vi "main.vi"() -> ()   [LabVIEW 2009]
panel:
  out "右表":dbl(knob) scale=0.0..100.0
  out "左表":dbl(knob) scale=0.0..100.0
  in  "右表旋转一圈":bool
  in  "stop":bool
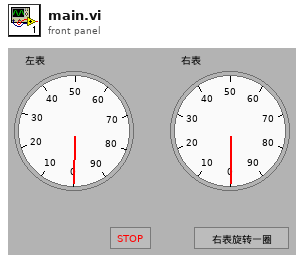
[diagram p1: front panel]
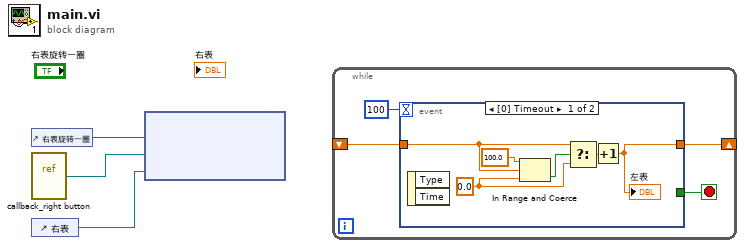
[diagram p0: block diagram]
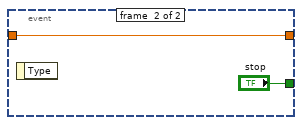
[diagram p2: hidden frame]
diagram:
  n1 = control-ref of="右表旋转一圈"() -> (w3:refnum<vi>)
  n2 = vi-ref "callback_right button.vi"() -> ("vi reference"=w1:refnum<vi>)
  n3 = control-ref of="右表"() -> (w2:refnum<vi>)
  n4 = node(w3, w1, w2) -> ()  [unwired: 2 in, 2 out]
  n5 = while {
    shift-right: [w5] -> _
    shift-left: _ -> [w6]
    stop <- w4 stop-if-true
    n6 = event shown="[0] Timeout" {
      selector: _ -> [_ _]
      dyn-events: _ -> [_ _]
      timeout: 100 -> [_ _]
      tunnel: w6 -> [w9 w14]
      tunnel: [w13 w14] -> w5
      tunnel: [_ "stop"] -> w4
      event #0 {
        w8 = 0.0 ("lower limit")
        n7 = event-data() -> ()  [unwired: 1 in, 2 out]
        n8 = In Range and Coerce(upper limit=100.0, x=w9, lower limit=w8) -> (In Range?=w11:bool)  [unwired: 1 out]
        n9 = Select(t=w9, s=w11, f=w8) -> (s? t:f=w10:dbl)
        n10 = Increment(x=w10) -> (x+1=w13:dbl)
        "左表" <- w13
      }
      event #1 {
        n11 = event-data() -> ()  [unwired: 1 in, 1 out]
      }
    }
  }
